vi "Parse Query.vi"(4 "Query String":string) -> (7 "Query Map":map{string, string}(c390))   [LabVIEW 2020, in "URI.lvlib"]
uses:
  URI.lvlib
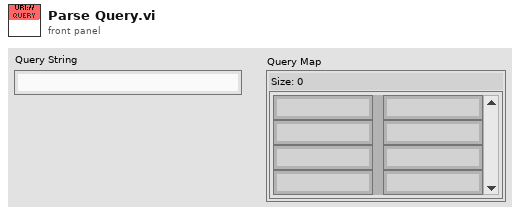
[diagram p1: front panel]
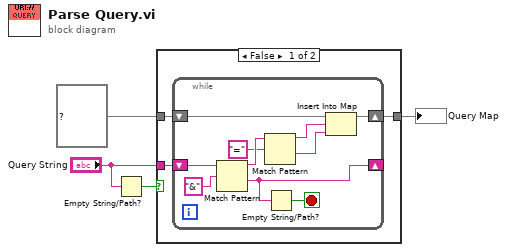
[diagram p0: block diagram]
diagram:
  n1 = Empty String/Path?(string/path="Query String") -> (empty?=w1:bool)
  n2 = case shown="False" w1 {
    tunnel: map{string, string} {} ("Query Map") -> [w7 w18]
    tunnel: [w6 w18] -> w3
    tunnel: "Query String" -> [w5 _]
    frame False {
      n3 = while {
        shift-right: [w9] -> _
        shift-left: w5 -> [w17]
        shift-right: [w10] -> w6
        shift-left: w7 -> [w13]
        stop <- w8 stop-if-true
        n4 = Match Pattern(string=w17, regular expression="&") -> (before substring=w15:string, after substring=w9:string)  [unwired: 1 in, 2 out]
        n5 = Match Pattern(string=w15, regular expression="=") -> (before substring=w12:string, after substring=w11:string)  [unwired: 1 in, 2 out]
        n6 = Empty String/Path?(string/path=w9) -> (empty?=w8:bool)
        n7 = Insert Into Map(map in=w13, key=w12, value=w11) -> (map out=w10:map{string, string})  [unwired: 2 out]
      }
    }
    frame True {
    }
  }
  "Query Map" <- w3
